vi "Counter with Load and Rollover and Variable Increment_2016.vi"(7 "Increment":u64, 8 "INC?":bool, 9 "Load Value":u64, 10 "Load?":bool) -> (3 "count":u64)   [LabVIEW 2016]
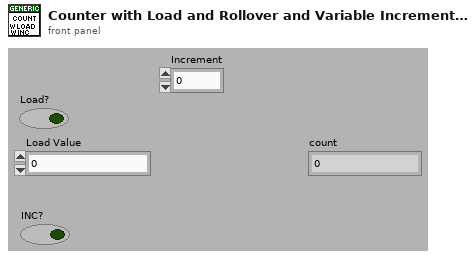
[diagram p1: front panel]
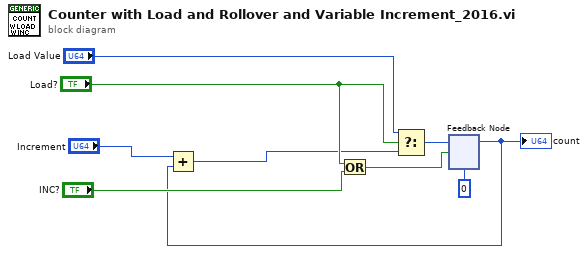
[diagram p0: block diagram]
diagram:
  n1 = Or(x="Load?", y="INC?") -> (x .or. y?=w4:bool)
  n2 = feedback #1(u64 0) -> (w3:u64)
  "count" <- w3
  n3 = Add(x="Increment", y=w3) -> (x+y=w2:u64)
  n4 = Select(t="Load Value", s="Load?", f=w2) -> (s? t:f=w5:u64)
  n5 = feedback-in #1(w5, w4) -> ()
